vi "AutoGen.vi"(8 "error in":errorcluster, 10 "References":T1) -> (0 "error out":errorcluster)   [LabVIEW 2014, in "UI Reference editor node.lvclass"]
doc: "Creates the tags for the channels an can create the tags based on the selected UI"
uses:
  UI Reference editor node.lvclass
  <vilib>/NI/DCAF/Tag Editor Core/Table API/Table Manager/object ref.ctl
  <vilib>/NI/DCAF/Tag Editor Core/Configuration Editor/Classes/Engine Parent/Engine Parent Editor Node.lvclass
  <vilib>/NI/DCAF/Tag Editor Core/Configuration Editor/Classes/Module editor node/module editor node.lvclass
  <vilib>/NI/Module Execution Interface/Engine Configuration/engine configuration.lvclass
  module/configuration/UI Reference configuration.lvclass
  module/configuration/Line.ctl
  <vilib>/NI/Tag Bus Module Framework/channel/TBM channel.lvclass
  <vilib>/NI/Configuration Framework/serializable configuration/NISE_CEF_serializable configuration.lvclass/NISE_CEF_serializable configuration.ctl
  <vilib>/Utility/LVClass/Get LV Class Name.vi
  <vilib>/NI/Configuration Framework/error generator/NISE_error generator.vi
  <vilib>/NI/Configuration Framework/serializable configuration/NISE_CEF_serializable configuration.lvclass
  <vilib>/NI/DCAF/Tag Editor Core/Table API/Table Manager/Table Manager.lvclass
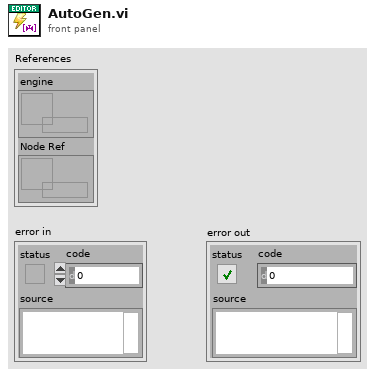
[diagram p1: front panel]
types:
  T1 = typedef "Table Manager.lvlib/Table Manager.lvclass/object ref.ctl" = cluster{"engine":refnum<data-value>, "Node Ref":refnum<data-value>}
  T2 = typedef "UI Reference configuration.lvclass/Line.ctl" = cluster{"channel":refnum<class "TBM channel.lvclass">}
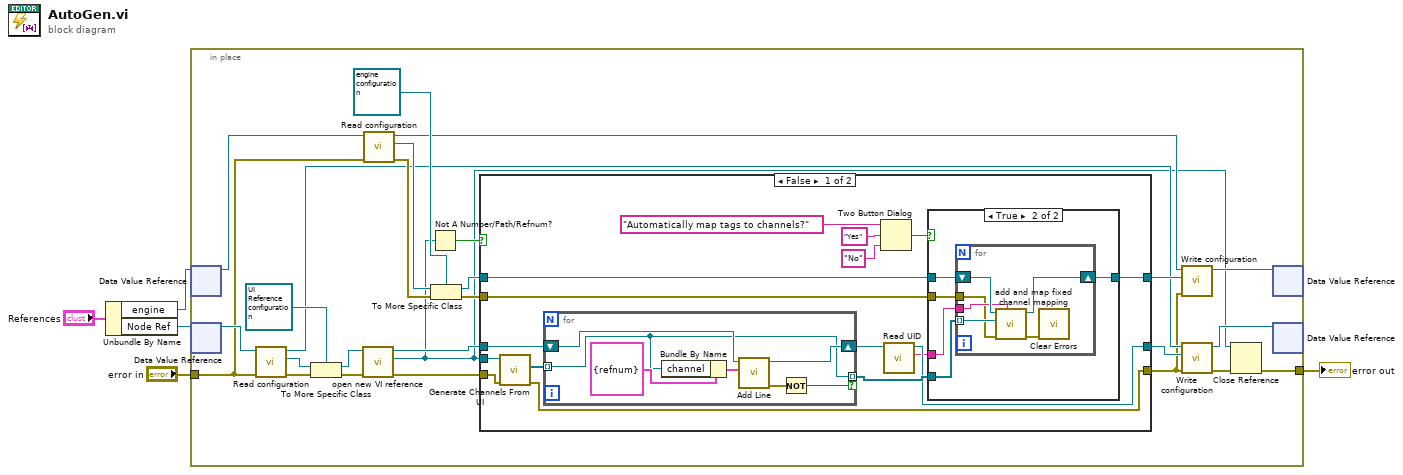
[diagram p0: block diagram]
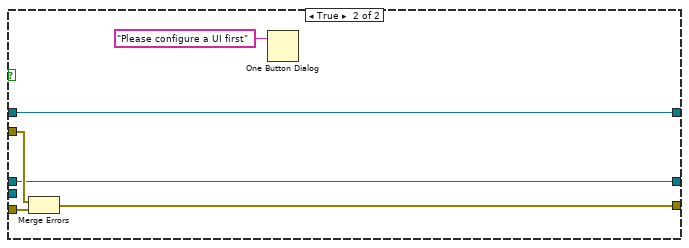
[diagram p3: hidden frame]
diagram:
  n1 = Unbundle By Name("References") -> ("engine"=w4:refnum<data-value>, "Node Ref"=w3:refnum<data-value>)
  n2 = in-place {
    in-place-border: [w7] -> w2
    in-place-border: "error in" -> [w6]
    n3 = in-place-dvr #1(w4) -> (w29:refnum<class "Engine Parent Editor Node.lvclass">)  [unwired: 1 out]
    n4 = in-place-dvr #2(w3) -> (w31:refnum<class "module editor node.lvclass">)  [unwired: 1 out]
    n5 = call-dynamic "Read configuration.vi"("error in"=w6, "NISE_CEF_serializable node in"=w31) -> ("error out"=w23:errorcluster, "configuration"=w30:refnum<class "NISE_CEF_serializable configuration.lvclass">, "NISE_CEF_serializable node out"=w19:refnum<class "module editor node.lvclass">)  [unwired: 7 in]
    n6 = To More Specific Class(target class=refnum<class "UI Reference configuration.lvclass"> refnum ("UI Reference configuration in"), reference=w30, error in=w23) -> (specific class reference=w11:refnum<class "UI Reference configuration.lvclass">, error out=w14:errorcluster)
    n7 = call "open new VI reference.vi"("error in"=w14, "UI Reference configuration"=w11) -> ("error out"=w13:errorcluster, "VI Refnum"=w8:refnum<vi>, "UI Reference configuration"=w12:refnum<class "UI Reference configuration.lvclass">)  [unwired: 7 in]
    n8 = call-dynamic "Read configuration.vi"("error in"=w6, "NISE_CEF_serializable node in"=w29) -> ("error out"=w26:errorcluster, "configuration"=w27:refnum<class "NISE_CEF_serializable configuration.lvclass">, "NISE_CEF_serializable node out"=w18:refnum<class "Engine Parent Editor Node.lvclass">)  [unwired: 7 in]
    n9 = Not A Number/Path/Refnum?(number/path/refnum=w8) -> (NaN/Path/Refnum?=w10:bool)
    n10 = To More Specific Class(target class=refnum<class "engine configuration.lvclass"> refnum ("engine configuration out"), reference=w27, error in=w26) -> (specific class reference=w25:refnum<class "engine configuration.lvclass">, error out=w22:errorcluster)
    n11 = case shown="False" w10 {
      tunnel: [w42 w72] -> w21
      tunnel: w25 -> [w43 w72]
      tunnel: [w39 w67] -> w20
      tunnel: [w37 w69] -> w15
      tunnel: w13 -> [w34 w70]
      tunnel: w22 -> [w35 w68]
      tunnel: w12 -> [w33 w67]
      tunnel: w8 -> [w32 _]
      frame False {
        n12 = call "Generate Channels From UI.vi"("error in"=w34, "VI Refnum"=w32) -> ("error out"=w37:errorcluster, "channels"=w36:refnum<class "TBM channel.lvclass">[])  [unwired: 8 in]
        n13 = for {
          tunnel: w36 -> [w60] mode=indexing
          shift-right: [w66] -> w44
          shift-left: w33 -> [w63]
          tunnel: [w60] -> w41 mode=indexing if=w64
          n14 = Bundle By Name(cluster=T2 {"channel"=refnum} ("Line"), "channel"=w60) -> (w61:T2)
          n15 = call "Add Line.vi"("Line"=w61, "UI Reference configuration in"=w63) -> ("error out"=w65:errorcluster, "UI Reference configuration out"=w66:refnum<class "UI Reference configuration.lvclass">)  [unwired: 7 in, 1 out]
          n16 = Not(x=w65) -> (.not. x?=w64:bool)
        }
        n17 = Two Button Dialog(message="Automatically map tags to channels?", 1:"No" ("F button name (\"Cancel\")"), 2:"Yes" ("T button name (\"OK\")")) -> (T button?=w45:bool)
        n18 = call <vilib>:"Read UID.vi"("configuration in"=w44) -> ("instance id"=w38:string, "configuration out"=w39:refnum<class "UI Reference configuration.lvclass">)  [unwired: 8 in, 1 out]
        n19 = case shown="True" w45 {
          tunnel: w43 -> [w48 w53]
          tunnel: [w48 w52] -> w42
          tunnel: w41 -> [_ w51]
          tunnel: w38 -> [_ w50]
          tunnel: w35 -> [_ w49]
          frame False {
          }
          frame True {
            n20 = for {
              shift-right: [w58] -> w52
              shift-left: w53 -> [w59]
              tunnel: w51 -> [w57] mode=indexing
              tunnel: w50 -> [w55]
              tunnel: w49 -> [w54]
              n21 = call <vilib>:"add and map fixed channel mapping.vi"("module instance"=w55, "error in"=w54, "fixed channel"=w57, "engine configuration in"=w59) -> ("error out"=w56:errorcluster, "engine configuration out"=w58:refnum<class "engine configuration.lvclass">)  [unwired: 6 in]
              n22 = call <vilib>:"Clear Errors.vi"("error in (no error)"=w56) -> ()  [unwired: 5 in, 2 out]
            }
          }
        }
      }
      frame True {
        n23 = Merge Errors(w68, w70) -> (w69:errorcluster)
        n24 = One Button Dialog(message="Please configure a UI first") -> ()  [unwired: 1 in, 1 out]
      }
    }
    n25 = call-dynamic "Write configuration.vi"("error in"=w15, "configuration"=w21, "NISE_CEF_serializable node in"=w18) -> ("NISE_CEF_serializable node out"=w17:refnum<class "Engine Parent Editor Node.lvclass">)  [unwired: 7 in, 1 out]
    n26 = call-dynamic "Write configuration.vi"("error in"=w15, "configuration"=w20, "NISE_CEF_serializable node in"=w19) -> ("error out"=w9:errorcluster, "NISE_CEF_serializable node out"=w16:refnum<class "module editor node.lvclass">)  [unwired: 7 in]
    n27 = Close Reference(reference=w8, error in (no error)=w9) -> (error out=w7:errorcluster)
    n28 = in-place-dvr #1(w17) -> ()  [unwired: 2 out]
    n29 = in-place-dvr #2(w16) -> ()  [unwired: 2 out]
  }
  "error out" <- w2
